vi "Convert array to image and save.vi"(1 "input array":dbl[][](array[numeric]), 2 "path to PNG file":path caption="PNG文件路径") -> ()   [LabVIEW 2021]
panel:
  out "x轴":i32
  out "y轴":i32
  out "Image display":dbl[][](graph)
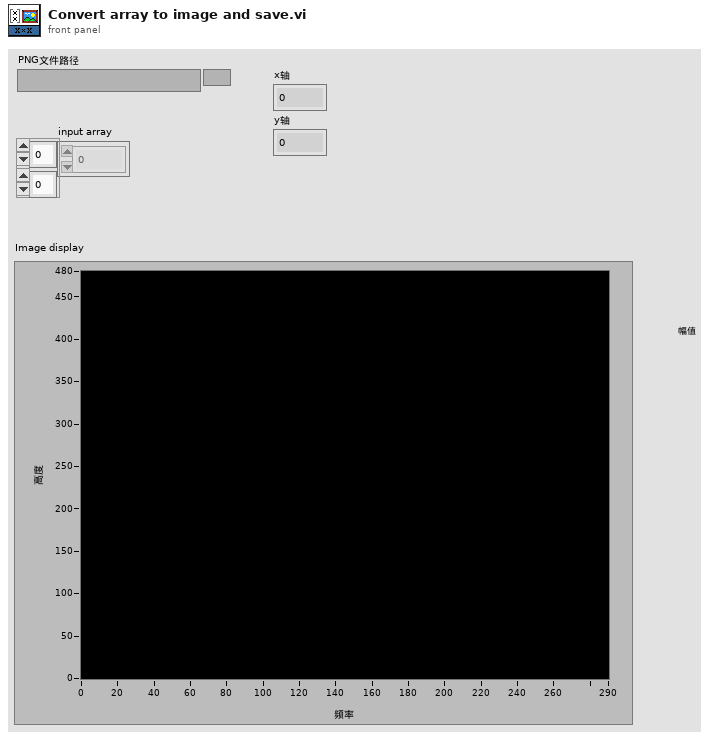
[diagram p1: front panel]
types:
  T1 = cluster{"image type":i32, "image type":i32, u8[], "mask":u8[], "mask":u32[], cluster{"索引":i16, "索引":i16, i16, i16}}
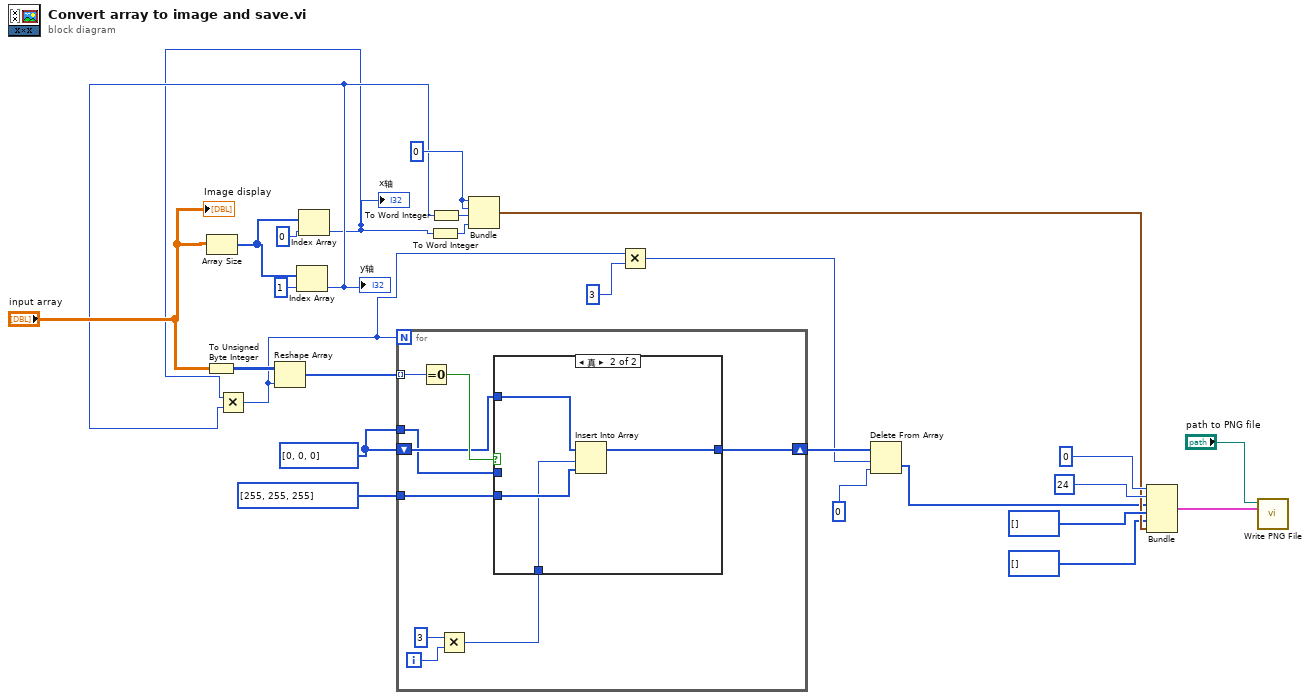
[diagram p0: block diagram]
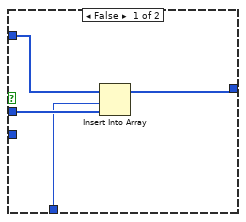
[diagram p2: hidden frame]
diagram:
  w15 = u8[] [0, 0, 0]
  w17 = i16 0 ("索引")
  n1 = To Unsigned Byte Integer(number="input array") -> (unsigned 8bit integer=w19:u8[][])
  n2 = Array Size(array="input array") -> (size(s)=w26:i32[])
  n3 = Index Array(array=w26, index=1 ("索引")) -> (element=w9:i32)
  "y轴" <- w9
  n4 = Index Array(array=w26, index=0 ("索引")) -> (element=w8:i32)
  "x轴" <- w8
  n5 = Multiply(x=w8, y=w9) -> (x*y=w3:i32)
  n6 = Reshape Array(w19, w3) -> (w12:u8[])
  n7 = for {
    N: w3 -> [_]
    tunnel: w12 -> [w35] mode=indexing
    tunnel: w15 -> [w30]
    tunnel: u8[] [255, 255, 255] -> [w33]
    shift-right: [w31] -> w6
    shift-left: w15 -> [w32]
    i -> [w29]
    n8 = Equal To 0?(x=w35) -> (x = 0?=w34:bool)
    n9 = Multiply(x=3, y=w29) -> (x*y=w27:i32)
    n10 = case shown="真" w34 {
      tunnel: w33 -> [_ w43]
      tunnel: w32 -> [w39 w42]
      tunnel: [w37 w41] -> w31
      tunnel: w30 -> [w38 _]
      tunnel: w27 -> [w36 w40]
      frame False {
        n11 = Insert Into Array(array=w39, index=w36, new element=w38) -> (w37:u8[])
      }
      frame True {
        n12 = Insert Into Array(array=w42, index=w40, new element=w43) -> (w41:u8[])
      }
    }
  }
  n13 = To Word Integer(number=w8) -> (16bit integer=w7:i16)
  n14 = To Word Integer(number=w9) -> (16bit integer=w10:i16)
  n15 = Bundle("索引"=w17, "索引"=w17, w10, w7) -> (w18:cluster{"索引":i16, "索引":i16, i16, i16})  [unwired: 1 in]
  n16 = Multiply(x=w3, y=3) -> (x*y=w1:i32)
  n17 = Delete From Array(array=w6, length=w1, index=0 ("索引")) -> (deleted portion=w5:u8[])  [unwired: 1 out]
  n18 = Bundle("image type"=0, "image type"=24, w5, "mask"=u8[] [], "mask"=u32[] [], w18) -> (w13:T1)  [unwired: 1 in]
  n19 = call <vilib>:"Write PNG File.vi"("image data"=w13, "path to PNG file"="path to PNG file") -> ()  [unwired: 8 in, 2 out]
  "Image display" <- "input array"
